vi "DDS RAM Programmer.vi"(6 "channel number (1)":u8=1 min=1 max=4 step=1, 7 "# of Words":u16, 8 "error in (no error)":errorcluster, 9 "RAM Destination":u8, 10 "RAM data":dbl[](array[numeric]), 11 "DDS ref in":T2={"NI USB-8451 device reference"="", "DIO port"=0, "Serial Clock Rate [kHz]"=1000}) -> (0 "error out":errorcluster, 2 "RAM data":u8[][](array[numeric]), 3 "DDS ref out":T2={"NI USB-8451 device reference"="", "DIO port"=0, "Serial Clock Rate [kHz]"=1000})   [LabVIEW 2013]
doc: "This VI sends the data from an array to the RAM memory of the DDS board. The correct profile needs to be selected by the PROFILE pins before executing this VI. Also the RAM Profiles should already be programmed so the DDS board knows where to store the data."
uses:
  DDS_box_device_reference.ctl
  <vilib>/ni845x/ni845x.llb/ni845xControl.ctl
  AD9910 registers.ctl
panel:
  in  "Channel Parameters":T1
  out "logical AND":bool
  out "RAM data check":u8[][](array[numeric])
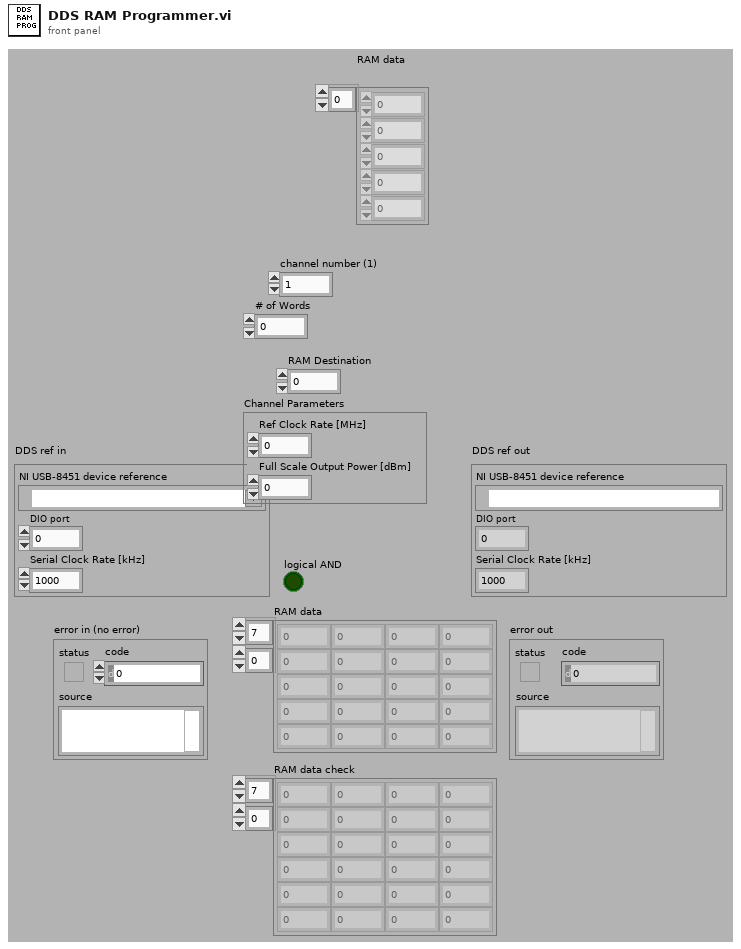
[diagram p1: front panel]
types:
  T1 = cluster{"Ref Clock Rate [MHz]":dbl, "Full Scale Output Power [dBm]":dbl}
  T2 = typedef "DDS_box_device_reference.ctl" = cluster{"NI USB-8451 device reference":T3, "DIO port":u8, "Serial Clock Rate [kHz]":u16}
  T3 = typedef "ni845xControl.ctl" = refnum<k21>
  T4 = typedef "AD9910 registers.ctl" = enum16{"CFR1", "CFR2", "CFR3", "Auxiliary DAC Control", "I/0 Update Rate", "Frequency Tuning Word", "Phase Offset Word", "Amplitude Scale Factor", "Multichip Sync", "Digital Ramp Limit", "Digital Ramp Step Size", "Digital Ramp Rate", "Single Tone Profile 0", "Single Tone Profile 1", "Single Tone Profile 2", "Single Tone Profile 3", "Single Tone Profile 4", "Single Tone Profile 5", "Single Tone Profile 6", "Single Tone Profile 7", "RAM Profile 0", "RAM Profile 1", "RAM Profile 2", "RAM Profile 3", "RAM Profile 4", "RAM Profile 5", "RAM Profile 6", "RAM Profile 7", "RAM"}
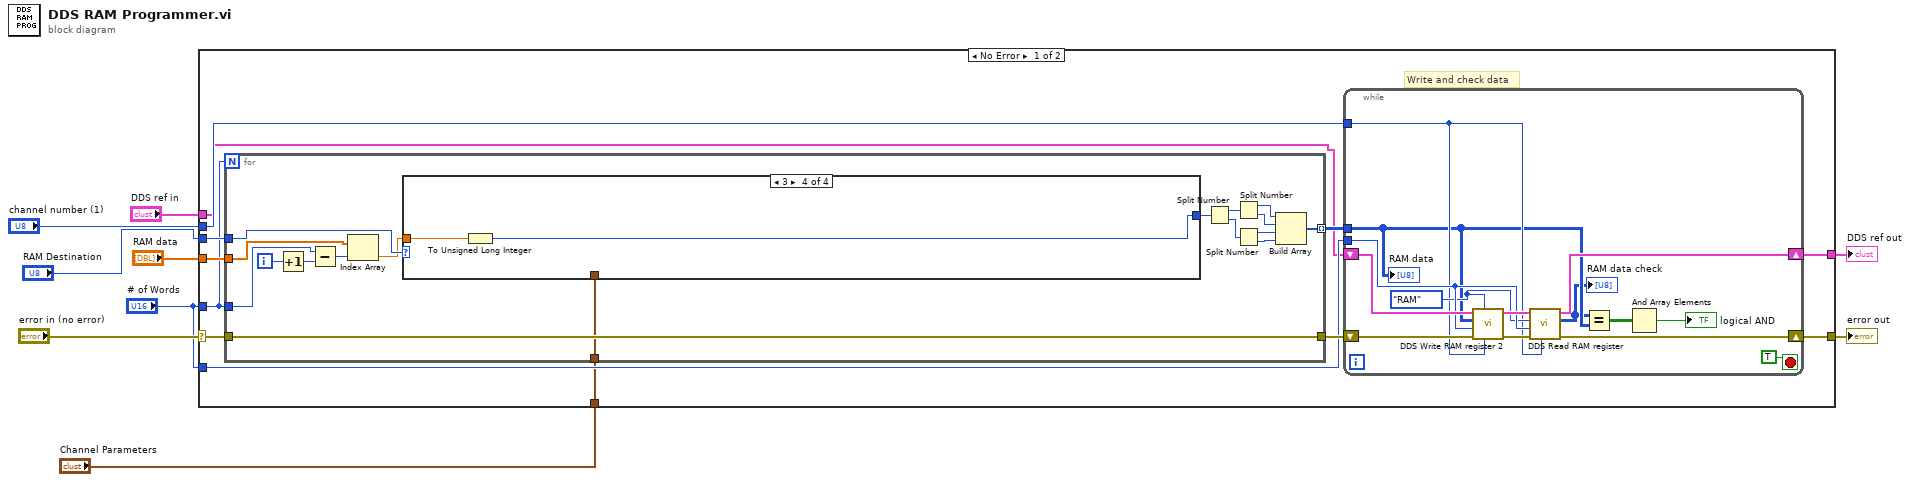
[diagram p0: block diagram]
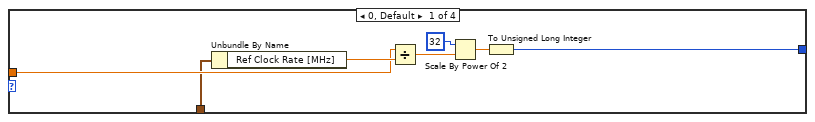
[diagram p2: hidden frame]
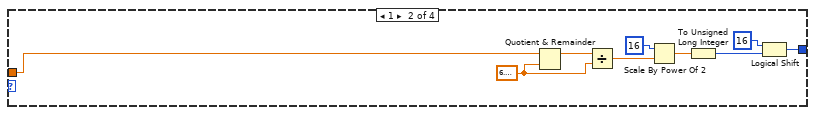
[diagram p3: hidden frame]
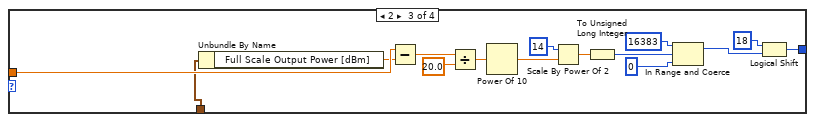
[diagram p4: hidden frame]
diagram:
  n1 = case shown="No Error" "error in (no error)" {
    selector: "error in (no error)" -> [w21 w86]
    tunnel: "DDS ref in" -> [w10 w87]
    tunnel: [w14 w86] -> w7
    tunnel: [w15 w87] -> w6
    tunnel: "RAM data" -> [w20 _]
    tunnel: "channel number (1)" -> [w16 _]
    tunnel: "RAM Destination" -> [w19 _]
    tunnel: "# of Words" -> [w17 _]
    tunnel: "# of Words" -> [w12 _]
    tunnel: "Channel Parameters" -> [w11 _]
    frame No Error {
      # "Write and check data"
      n2 = for {
        N: w12 -> [_]
        tunnel: w21 -> [w44]
        tunnel: [w44] -> w18
        tunnel: w20 -> [w41]
        tunnel: w19 -> [w46]
        tunnel: [w43] -> w13 mode=indexing
        tunnel: w12 -> [w37]
        tunnel: w11 -> [w36]
        i -> [w39]
        n3 = Increment(x=w39) -> (x+1=w38:i32)
        n4 = Subtract(x=w37, y=w38) -> (x-y=w40:i32)
        n5 = Index Array(array=w41, index=w40) -> (element=w45:dbl)
        n6 = case shown="3" w46 {
          tunnel: w45 -> [w54 w63 w77 w85]
          tunnel: [w55 w61 w72 w84] -> w42
          tunnel: w36 -> [w53 _ w69 _]
          frame 0, Default {
            n7 = Unbundle By Name(w53) -> ("Ref Clock Rate [MHz]"=w56:dbl)
            n8 = Divide(x=w54, y=w56) -> (x/y=w59:dbl)
            n9 = Scale By Power Of 2(n=32 ("x"), x=w59) -> (x*2^n=w57:dbl)
            n10 = To Unsigned Long Integer(number=w57) -> (unsigned 32bit integer=w55:u32)
          }
          frame 1 {
            w64 = 6.283185307179586
            n11 = Quotient & Remainder(x=w63, y=w64) -> (x-y*floor(x/y)=w67:dbl)  [unwired: 1 out]
            n12 = Divide(x=w67, y=w64) -> (x/y=w65:dbl)
            n13 = Scale By Power Of 2(n=16, x=w65) -> (x*2^n=w66:dbl)
            n14 = To Unsigned Long Integer(number=w66) -> (unsigned 32bit integer=w62:u32)
            n15 = Logical Shift(y=i8 16, x=w62) -> (x << y=w61:u32)
          }
          frame 2 {
            n16 = Unbundle By Name(w69) -> ("Full Scale Output Power [dBm]"=w76:dbl)
            n17 = Subtract(x=w77, y=w76) -> (x-y=w83:dbl)
            n18 = Divide(x=w83, y=20.0) -> (x/y=w81:dbl)
            n19 = Power Of 10(x=w81) -> (10^x=w80:dbl)
            n20 = Scale By Power Of 2(n=14, x=w80) -> (x*2^n=w78:dbl)
            n21 = To Unsigned Long Integer(number=w78) -> (unsigned 32bit integer=w73:u32)
            n22 = In Range and Coerce(upper limit=u32 16383, x=w73, lower limit=u32 0) -> (coerced(x)=w71:u32)  [unwired: 1 out]
            n23 = Logical Shift(y=i8 18, x=w71) -> (x << y=w72:u32)
          }
          frame 3 {
            n24 = To Unsigned Long Integer(number=w85) -> (unsigned 32bit integer=w84:u32)
          }
        }
        n25 = Split Number(x=w42) -> (hi(x)=w52:u16, lo(x)=w51:u16)
        n26 = Split Number(x=w52) -> (hi(x)=w47:u8, lo(x)=w48:u8)
        n27 = Split Number(x=w51) -> (hi(x)=w49:u8, lo(x)=w50:u8)
        n28 = Build Array(w47, w48, w49, w50) -> (w43:u8[])
      }
      n29 = while {
        tunnel: w17 -> [w31]
        tunnel: w16 -> [w29]
        tunnel: w13 -> [w26]
        shift-right: [w28] -> w15
        shift-left: w10 -> [w35]
        shift-right: [w27] -> w14
        shift-left: w18 -> [w34]
        stop <- TRUE stop-if-true
        w30 = AD9910_registers."RAM" ("Register")
        n30 = call "DDS Write RAM register 2.vi"("channel number (1)"=w29, "Register"=w30, "error in (no error)"=w34, "# of Words"=w31, "Write Data"=w26, "DDS ref in"=w35) -> ("error out"=w32:errorcluster, "DDS ref out"=w33:T2)  [unwired: 4 in]
        n31 = call "DDS Read RAM register.vi"("channel number (1)"=w29, "error in (no error)"=w32, "# of Words"=w31, "Register"=w30, "DDS ref in"=w33) -> ("error out"=w27:errorcluster, "RAM data"=w24:u8[][], "DDS ref out"=w28:T2)  [unwired: 4 in]
        "RAM data check" <- w24
        n32 = Equal?(x=w24, y=w26) -> (x = y?=w25:bool[][])
        n33 = And Array Elements(Boolean array=w25) -> (logical AND=→"logical AND":bool)
        "RAM data" <- w26
      }
    }
    frame Error {
    }
  }
  "error out" <- w7
  "DDS ref out" <- w6
